vi "juntar 5 medidas.vi"() -> ()   [LabVIEW 2021]
uses:
  <vilib>/Analysis/1siggen.llb/Ramp Pattern by Delta.vi
  <vilib>/Analysis/NI_AAL_SigProc.lvlib
  <vilib>/Analysis/NI_AALPro.lvlib
  <vilib>/Analysis/NI_AALBase.lvlib
panel:
  out "Histogram Graph 3":T1(graph)
  out "Histogram Graph 2":T2(graph)
  out "Curva de potencia":cluster{"Ramp Pattern":dbl[], dbl[]}(graph)
  out "Pulsos totales":i32
  out "Histogram Graph":T2
  in  "# bins":i32
  in  "min":dbl format="%0.2f"
  in  "max":dbl format="%0.2f"
  in  "threshold":dbl format="%0.2f"
  in  "Filename 5":path=path "test.lvm" caption="Filename"
  in  "Filename 4":path=path "test.lvm" caption="Filename"
  in  "Filename 3":path=path "test.lvm" caption="Filename"
  in  "Filename 2":path=path "test.lvm" caption="Filename"
  in  "Filename":path=path "test.lvm"
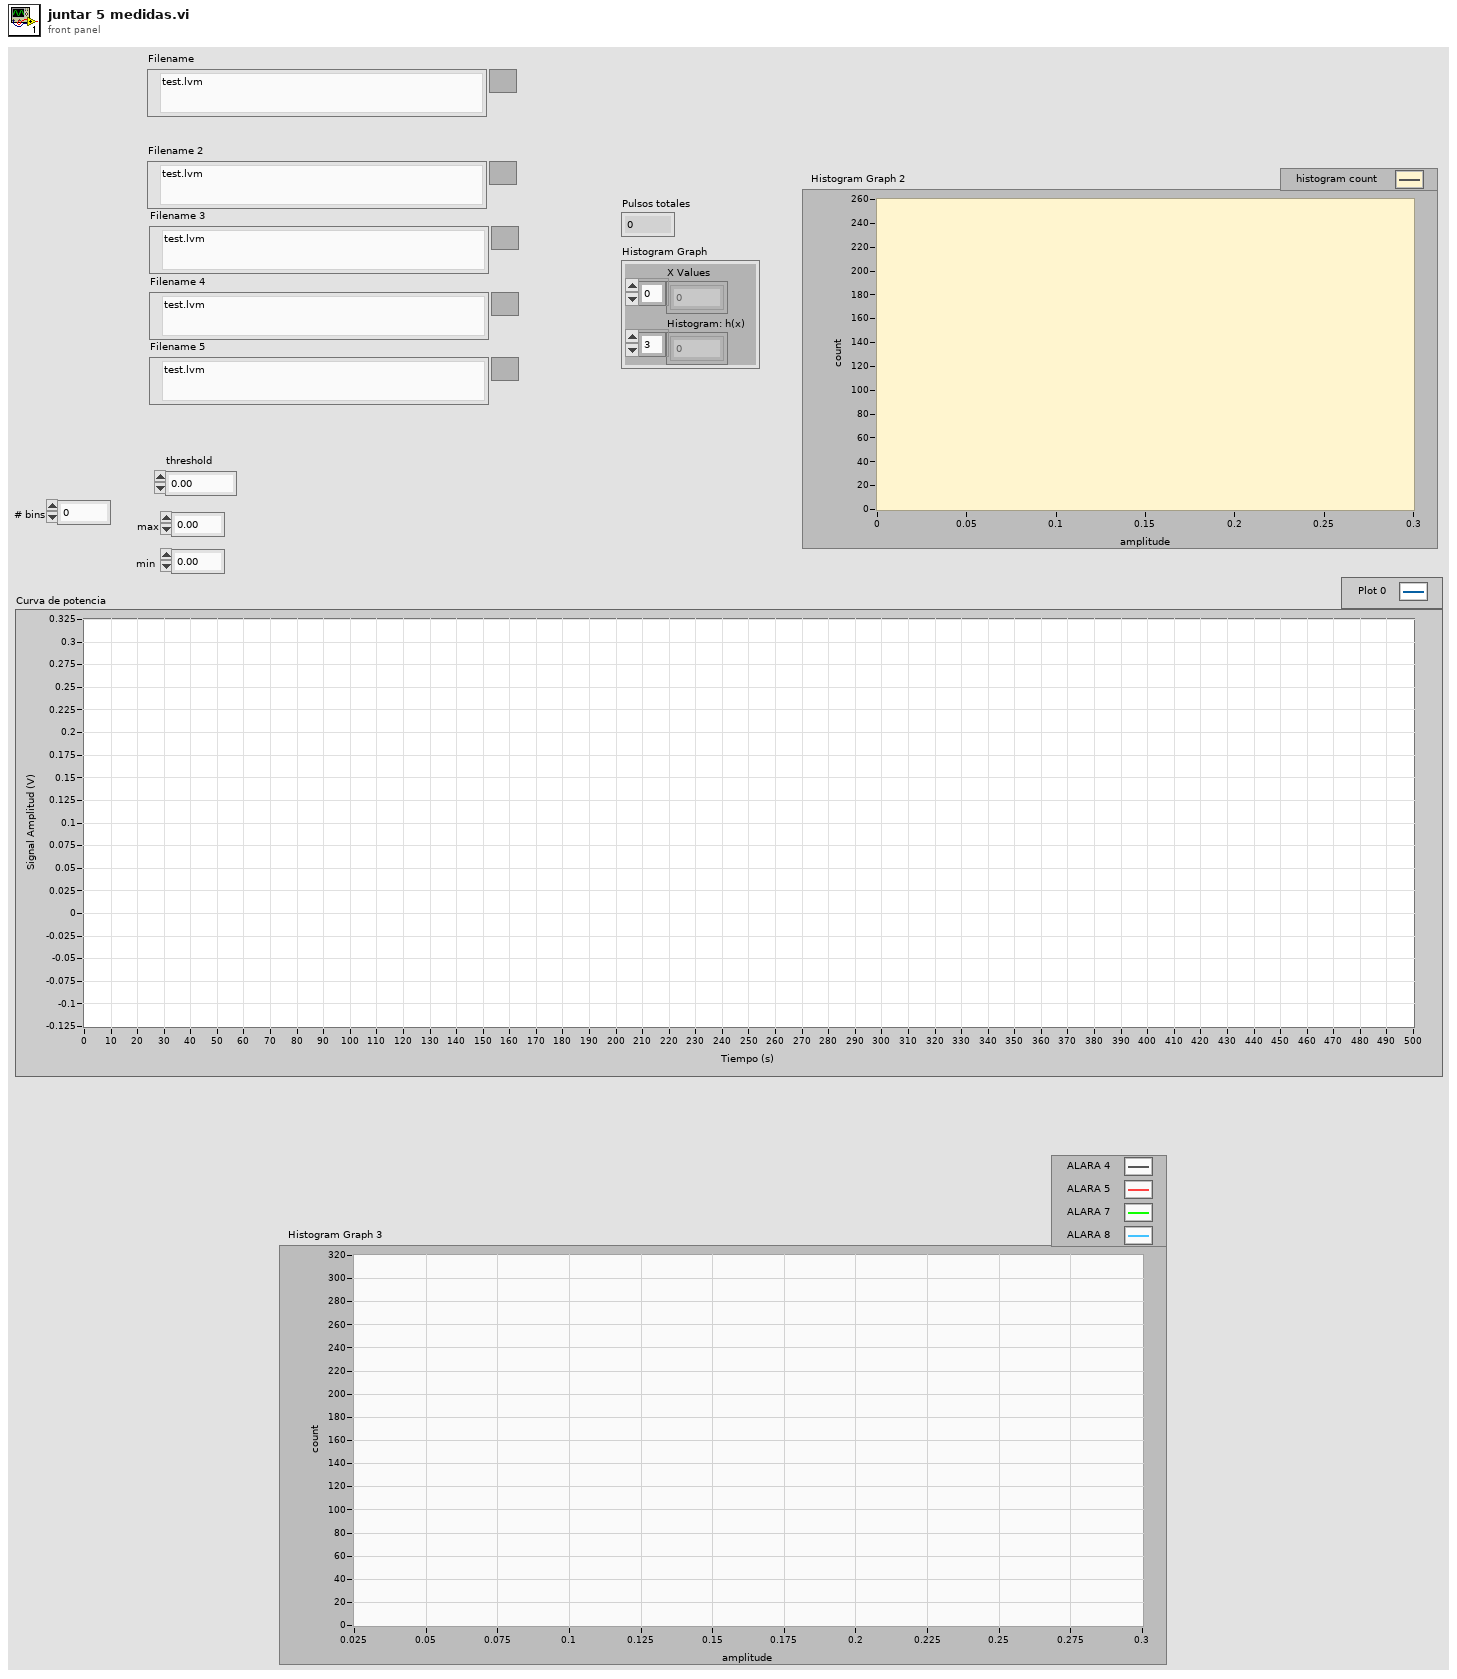
[diagram p1: front panel]
types:
  T1 = cluster{"X Values":dbl[], "Histogram: h(x)":i32[]}[]
  T2 = cluster{"X Values":dbl[], "Histogram: h(x)":i32[]}
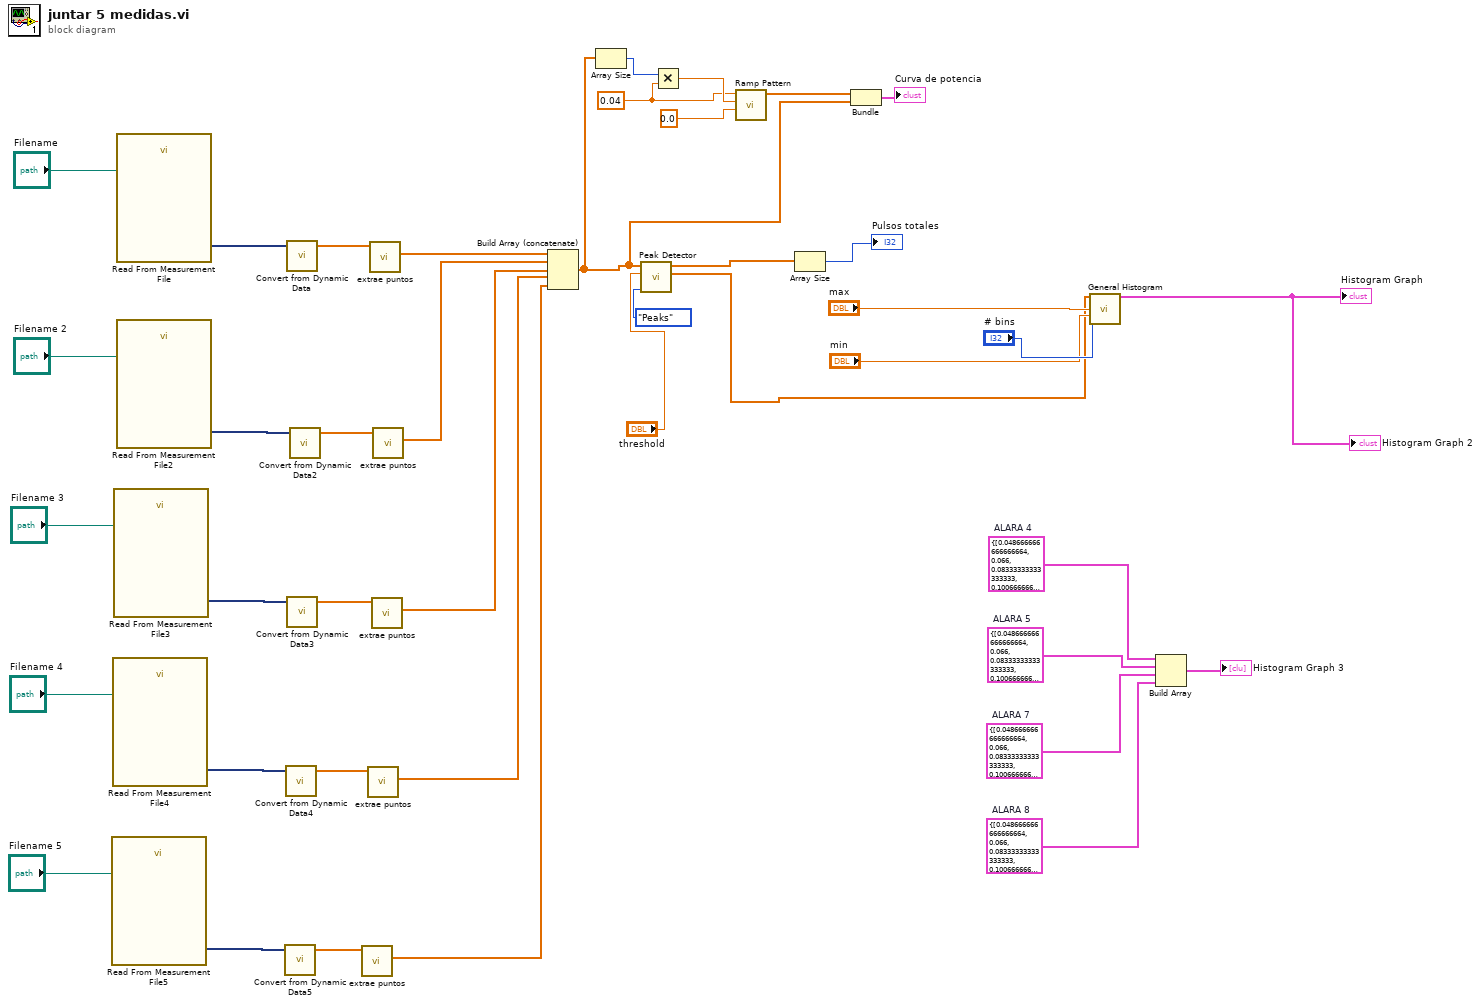
[diagram p0: block diagram]
diagram:
  w2 = T2 {"X Values"=[0.048666666666666664, 0.066, 0.08333333333333333, 0.10066666666666667, 0.11800000000000001, 0.13533333333333333, 0.15266666666666667, 0.16999999999999998, 0.18733333333333335, 0.20466666666666666, 0.222, 0.23933333333333334, 0.25666666666666665, 0.27399999999999997, 0.29133333333333333], "Histogram: h(x)"=[297, 99, 78, 66, 52, 33, 28, 14, 12, 12, 4, 5, 3, 0, 1]}  # ALARA 8
  w3 = T2 {"X Values"=[0.048666666666666664, 0.066, 0.08333333333333333, 0.10066666666666667, 0.11800000000000001, 0.13533333333333333, 0.15266666666666667, 0.16999999999999998, 0.18733333333333335, 0.20466666666666666, 0.222, 0.23933333333333334, 0.25666666666666665, 0.27399999999999997, 0.29133333333333333], "Histogram: h(x)"=[255, 96, 100, 57, 28, 34, 35, 25, 14, 8, 7, 9, 3, 0, 1]}  # ALARA 7
  w4 = T2 {"X Values"=[0.048666666666666664, 0.066, 0.08333333333333333, 0.10066666666666667, 0.11800000000000001, 0.13533333333333333, 0.15266666666666667, 0.16999999999999998, 0.18733333333333335, 0.20466666666666666, 0.222, 0.23933333333333334, 0.25666666666666665, 0.27399999999999997, 0.29133333333333333], "Histogram: h(x)"=[277, 95, 49, 50, 32, 33, 19, 24, 12, 11, 2, 5, 4, 2, 0]}  # ALARA 5
  w5 = T2 {"X Values"=[0.048666666666666664, 0.066, 0.08333333333333333, 0.10066666666666667, 0.11800000000000001, 0.13533333333333333, 0.15266666666666667, 0.16999999999999998, 0.18733333333333335, 0.20466666666666666, 0.222, 0.23933333333333334, 0.25666666666666665, 0.27399999999999997, 0.29133333333333333], "Histogram: h(x)"=[317, 91, 64, 72, 48, 39, 29, 17, 9, 9, 3, 2, 1, 1, 1]}  # ALARA 4
  w11 = 0.04 ("end")
  n1 = call "Read From Measurement File5"("Filename"="Filename 5") -> ("Signals"=w32:dynamicdata)  [unwired: 5 in, 5 out]
  n2 = call "Read From Measurement File4"("Filename"="Filename 4") -> ("Signals"=w35:dynamicdata)  [unwired: 5 in, 5 out]
  n3 = call "Read From Measurement File3"("Filename"="Filename 3") -> ("Signals"=w36:dynamicdata)  [unwired: 5 in, 5 out]
  n4 = call "Read From Measurement File"("Filename"="Filename") -> ("Signals"=w40:dynamicdata)  [unwired: 5 in, 5 out]
  n5 = call "Read From Measurement File2"("Filename"="Filename 2") -> ("Signals"=w39:dynamicdata)  [unwired: 5 in, 5 out]
  n6 = call "Convert from Dynamic Data5"("Dynamic Data Type"=w32) -> ("Array"=w30:dbl[])  [unwired: 3 in]
  n7 = call "Convert from Dynamic Data4"("Dynamic Data Type"=w35) -> ("Array"=w29:dbl[])  [unwired: 3 in]
  n8 = call "Convert from Dynamic Data"("Dynamic Data Type"=w40) -> ("Array"=w31:dbl[])  [unwired: 3 in]
  n9 = call "Convert from Dynamic Data3"("Dynamic Data Type"=w36) -> ("Array"=w28:dbl[])  [unwired: 3 in]
  n10 = call "Convert from Dynamic Data2"("Dynamic Data Type"=w39) -> ("Array"=w27:dbl[])  [unwired: 3 in]
  n11 = call "extrae puntos.vi"("Array in"=w30) -> ("Array out"=w22:dbl[])  [unwired: 8 in, 2 out]
  n12 = call "extrae puntos.vi"("Array in"=w29) -> ("Array out"=w23:dbl[])  [unwired: 8 in, 2 out]
  n13 = call "extrae puntos.vi"("Array in"=w31) -> ("Array out"=w26:dbl[])  [unwired: 8 in, 2 out]
  n14 = call "extrae puntos.vi"("Array in"=w28) -> ("Array out"=w24:dbl[])  [unwired: 8 in, 2 out]
  n15 = call "extrae puntos.vi"("Array in"=w27) -> ("Array out"=w25:dbl[])  [unwired: 8 in, 2 out]
  n16 = Build Array (concatenate)(w26, w25, w24, w23, w22) -> (w7:dbl[])
  n17 = Array Size(array=w7) -> (size(s)=w8:i32)
  n18 = call <vilib>:"Peak Detector.vi"("peaks/valleys"=enum32{"Peaks", "Valleys"}."Peaks", "threshold"="threshold", "X"=w7) -> ("Amplitudes"=w18:dbl[], "Locations"=w17:dbl[])  [unwired: 4 in, 3 out]
  n19 = Multiply(x=w8, y=w11) -> (x*y=w12:dbl)
  n20 = call-poly <vilib>:"Ramp Pattern.vi"("start"=0.0 ("end"), "end"=w12, "delta"=w11) -> ("Ramp Pattern"=w10:dbl[])  [unwired: 6 in, 2 out]
  n21 = Array Size(array=w17) -> (size(s)=→"Pulsos totales":i32)
  n22 = Bundle("Ramp Pattern"=w10, w7) -> (→"Curva de potencia":cluster{"Ramp Pattern":dbl[], dbl[]})  [unwired: 1 in]
  n23 = call <vilib>:"General Histogram.vi"("X"=w18, "max"="max", "min"="min", "# bins"="# bins") -> ("Histogram Graph"=→"Histogram Graph" →"Histogram Graph 2":T2)  [unwired: 7 in, 4 out]
  n24 = Build Array(w5, w4, w3, w2) -> (→"Histogram Graph 3":T1)
